vi "GalvosInitialize.vi"(6 "Cursor Position (V)":cluster{"Cursor X":dbl, "Cursor Y":dbl}, 8 "error in (no error)":errorcluster, 11 "Microscope in":refnum<class "Microscope.lvclass">) -> (0 "error out":errorcluster, 1 "Galvo Write Rate":dbl, 2 "actual write rate":dbl, 3 "Microscope out":refnum<class "Microscope.lvclass">, 4 "Galvo Timebase divisor":i32)   [LabVIEW 2012, in "Microscope.lvclass"]
uses:
  classes/Microscope.lvclass
  classes/Microscope.lvclass/Microscope.ctl
  <vilib>/DAQmx/write.llb/DAQmx Write (Analog 1D Wfm NChan NSamp).vi
  <vilib>/DAQmx/create/channels.llb/DAQmx Create Channel (AO-Voltage-Basic).vi
  <vilib>/DAQmx/configure/timing.llb/DAQmx Timing (Sample Clock).vi
  <vilib>/DAQmx/configure/trigger.llb/DAQmx Start Trigger (Digital Edge).vi
  <vilib>/DAQmx/miscellaneous.llb/DAQmx Fill In Error Info.vi
  <resource>/objmgr/daqmx.rc
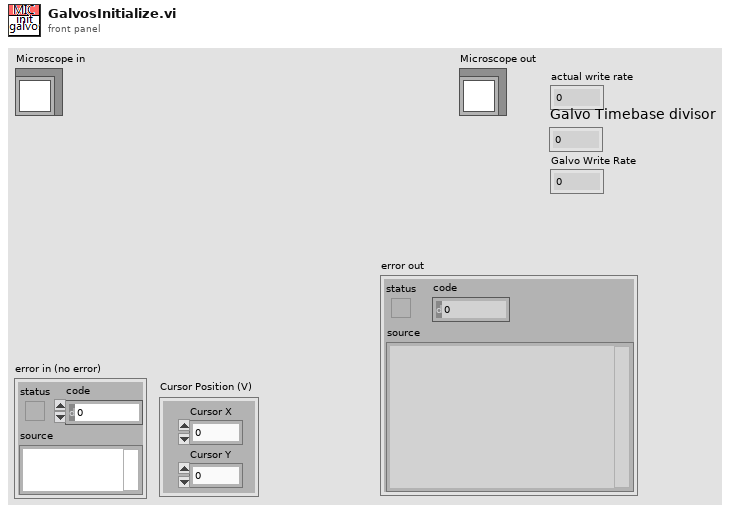
[diagram p1: front panel]
types:
  T1 = typedef "Scan Type.ctl" = enum16{"None", "Point", "Full Image Continuous", "Full Image Grab"}
  T2 = typedef "SyncAlgo.ctl" = cluster{"Pixels/sec":dbl, "Pixel Dwell Time (us)":dbl, "Fill Factor":dbl, "Flyback Pixels":dbl, "Lines/sec":dbl, "Galvo Write rate":dbl, "Galvo Timebase divisor":i32, "total pixels per line":dbl, "Samples to Average":dbl, "Trash Samples":dbl, "Actual samples to Read per Line":dbl, "Detector Read rate":dbl, "Detector Timebase divisor":i32}
  T3 = cluster{"x pixels":i32, "x voltage min":dbl, "x voltage max":dbl, "y pixels":i32, "y voltage min":dbl, "y voltage max":dbl, "x pts flyback":i32, "y pts flyback":i32, "Zoom":dbl}
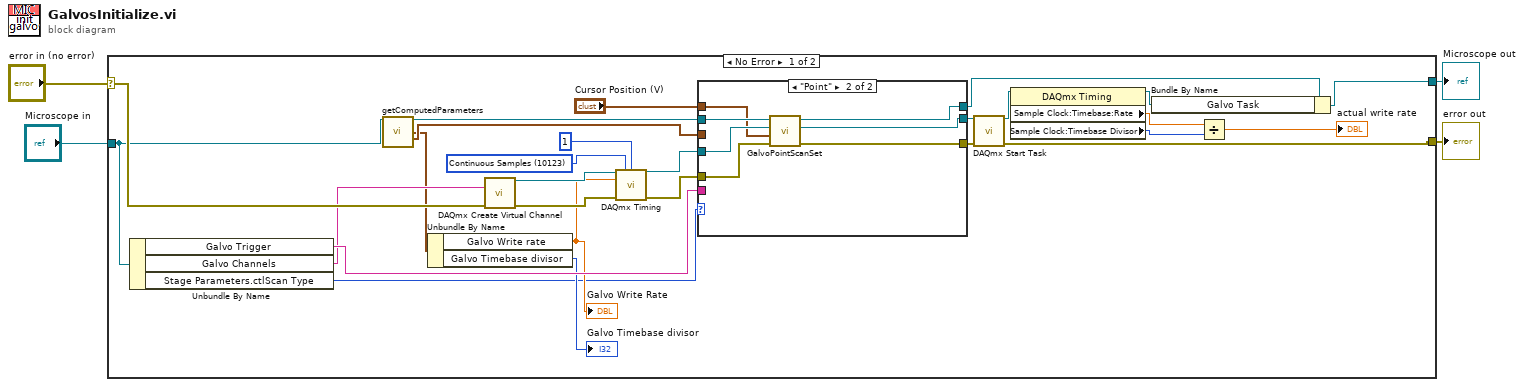
[diagram p0: block diagram]
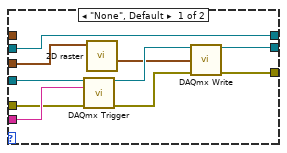
[diagram p2: hidden frame]
diagram:
  n1 = case shown="No Error" "error in (no error)" {
    selector: "error in (no error)" -> [w30 w50]
    tunnel: [w29 w50] -> w3
    tunnel: [w31 w49] -> w1
    tunnel: "Microscope in" -> [w28 w49]
    frame No Error {
      w24 = 10123 items=["Finite Samples"=10178, "Continuous Samples"=10123, "Hardware Timed Single Point"=12522] ("sample mode")
      n2 = Unbundle By Name(w28) -> ("Galvo Trigger"=w27:tag, "Galvo Channels"=w26:tag, "Stage Parameters.ctlScan Type"=w5:T1)
      n3 = call "getComputedParameters.vi"("Microscope in"=w28) -> ("Microscope out"=w8:refnum<class "Microscope.lvclass">, "Computed Parameters"=w11:T2, "Scanning Parameters"=w12:T3)  [unwired: 11 in, 1 out]
      n4 = Unbundle By Name(w11) -> ("Galvo Write rate"=w10:dbl, "Galvo Timebase divisor"=→"Galvo Timebase divisor":i32)
      "Galvo Write Rate" <- w10
      n5 = call-poly <vilib>:"DAQmx Create Virtual Channel.vi"("physical channels"=w26, "error in"=w30) -> ("task out"=w25:refnum<k21>, "error out"=w22:errorcluster)  [unwired: 12 in]
      n6 = call-poly <vilib>:"DAQmx Timing.vi"("task/channels in"=w25, "sample mode"=w24, "samples per channel"=1, "rate"=w10, "error in"=w22) -> ("task out"=w23:refnum<k21>, "error out"=w21:errorcluster)  [unwired: 9 in]
      n7 = case shown="\"Point\"" w5 {
        tunnel: w27 -> [w41 _]
        tunnel: w23 -> [w40 w46]
        tunnel: w21 -> [w37 w45]
        tunnel: [w35 w48] -> w20
        tunnel: [w34 w47] -> w13
        tunnel: w12 -> [w33 _]
        tunnel: w8 -> [w32 w44]
        tunnel: [w32 w43] -> w7
        tunnel: "Cursor Position (V)" -> [_ w42]
        frame "None", Default {
          n8 = call-poly <vilib>:"DAQmx Trigger.vi"("task/channels in"=w40, "source"=w41, "error in"=w37) -> ("task out"=w39:refnum<k21>, "error out"=w36:errorcluster)  [unwired: 11 in]
          n9 = call "2D raster.vi"("Scanning Parameters"=w33) -> ("X and Y"=w38:waveform(dbl)[])  [unwired: 8 in, 2 out]
          n10 = call-poly <vilib>:"DAQmx Write.vi"("task/channels in"=w39, "data"=w38, "error in"=w36) -> ("task out"=w34:refnum<k21>, "error out"=w35:errorcluster)  [unwired: 10 in, 1 out]
        }
        frame "Point" {
          n11 = call "GalvoPointScanSet.vi"("error in (no error)"=w45, "Cursor Position (V)"=w42, "task in"=w46, "Microscope in"=w44) -> ("error out"=w48:errorcluster, "task out"=w47:refnum<k21>, "Microscope out"=w43:refnum<class "Microscope.lvclass">)  [unwired: 5 in]
        }
      }
      n12 = call <vilib>:"DAQmx Start Task.vi"("task/channels in"=w13, "error in"=w20) -> ("task out"=w14:refnum<k21>, "error out"=w29:errorcluster)  [unwired: 12 in]
      n13 = property class="DAQmx Timing"(reference=w14) -> (reference out=w18:refnum<k21>, "Sample Clock:Timebase:Rate"=w17:dbl, "Sample Clock:Timebase Divisor"=w16:u32)  [unwired: 1 in, 1 out]
      n14 = Bundle By Name(cluster=w7, "Galvo Task"=w18) -> (w31:refnum<class "Microscope.lvclass">)
      n15 = Divide(x=w17, y=w16) -> (x/y=→"actual write rate":dbl)
    }
    frame Error {
    }
  }
  "error out" <- w3
  "Microscope out" <- w1
